vi "Server Panel.vi"(8 "error in":errorcluster, 11 "server session ref":variant) -> (0 "error out":errorcluster, 3 "server session ref out":variant)   [LabVIEW 2020]
doc: "This is panel of TWM server. When the server is running, a client can connect to the created named pipe and control some of the TWM function via the pipe. This panel must be opened to keep the server alive!"
uses:
  Server Session Reference.ctl
  Server Session.ctl
  varilib/SGUI Assign References Mode.ctl
  Server Event.ctl
  Server Client Request.ctl
  Server Event Command.ctl
  varilib/SGUI Assign Multiple Strings With Tags By Label.vi
  varilib/varilib.lvlib
panel:
  out "log panel ref":refnum<vi>
  out "log ref":refnum<vi>
  in  "btn view log":bool
  in  "Log traffic":bool
  out "srv session":T1
  out "server":i32
  in  "btn srv exit":bool
  out "str last cmd":string caption="Last command header"
  out "led run":bool caption="Running"
  in  "btn srv stop":bool
  in  "btn srv start":bool
  in  "pipe name":string="\\\\.\\pipe\\TWM:server" caption="Named Pipe Identifier"
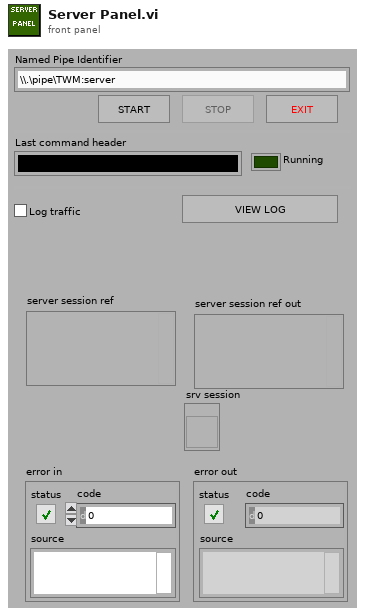
[diagram p1: front panel]
types:
  T1 = typedef "Server Session Reference.ctl" = refnum<vi>
  T2 = typedef "varilib.lvlib/SGUI Assign References Mode.ctl" = enum16{"Add to stack", "Overwrite", "Release last", "Release ID"}
  T3 = typedef "Server Session.ctl" = cluster{"cmd event":variant, "answer event":variant}
  T4 = typedef "Server Event.ctl" = cluster{"client request":T5, "command":T6}
  T5 = typedef "Server Client Request.ctl" = cluster{"info data":string, "answer handle":i32}
  T6 = typedef "Server Event Command.ctl" = enum16{"None", "Restart", "Identify", "Set measurement", "Start", "Get status", "Get result", "Stop", "Set corrections", "Get algorithm info"}
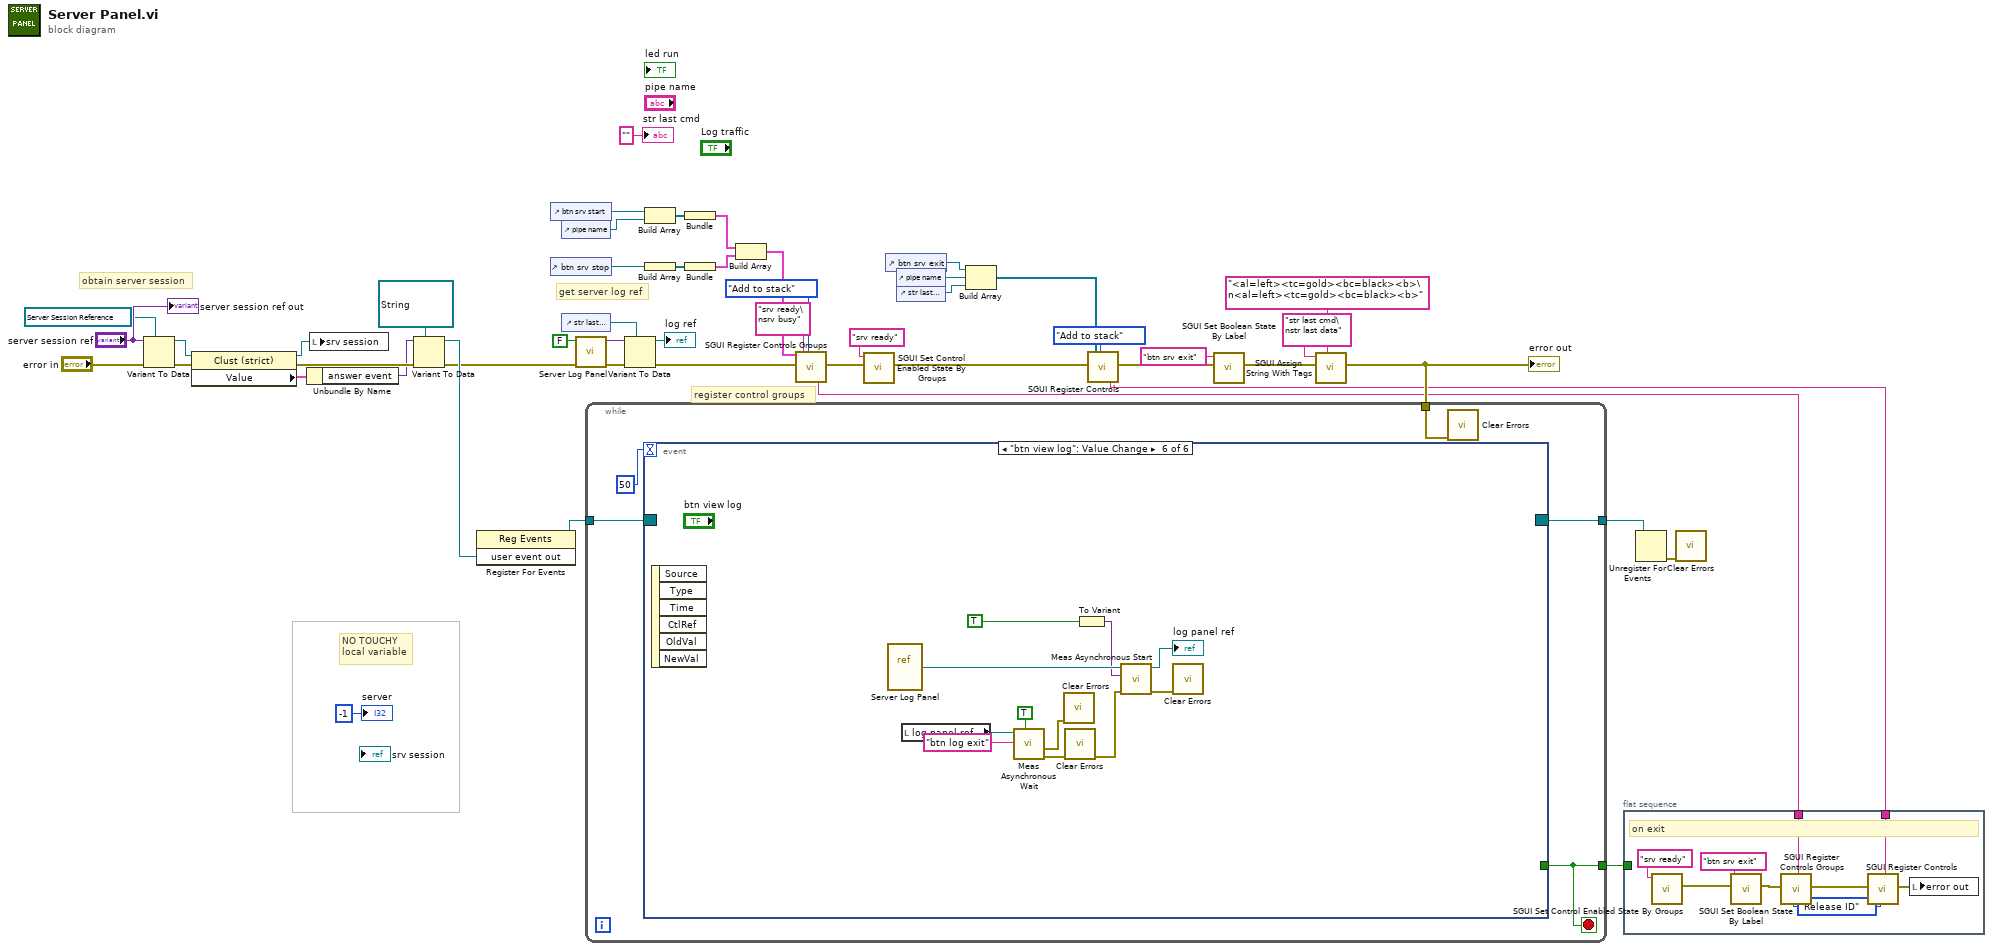
[diagram p0: block diagram]
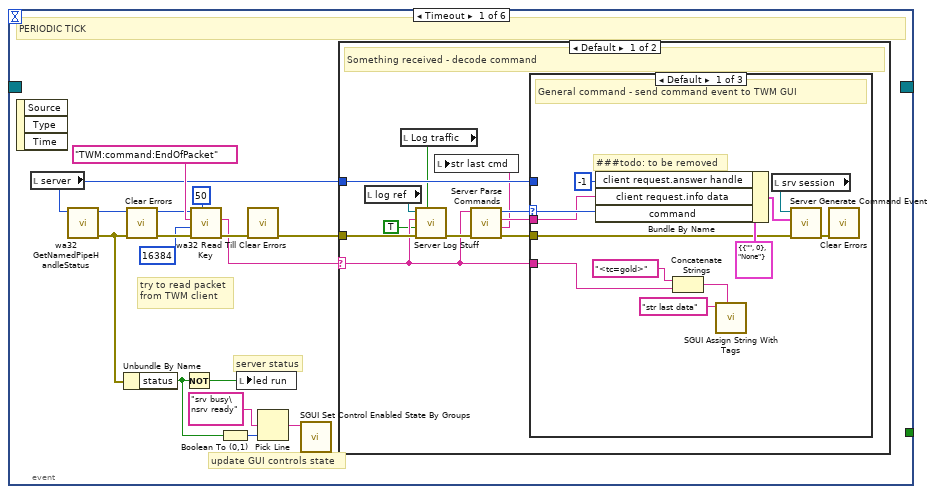
[diagram p2: hidden frame]
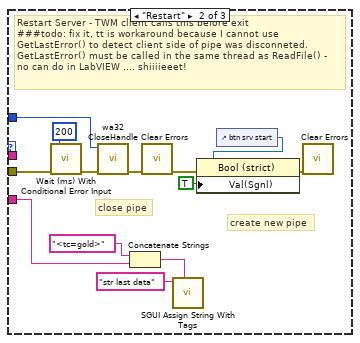
[diagram p3: hidden frame]
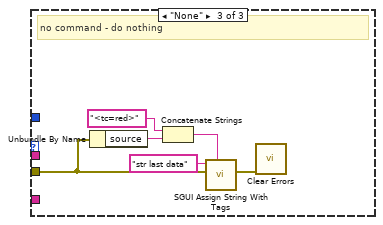
[diagram p4: hidden frame]
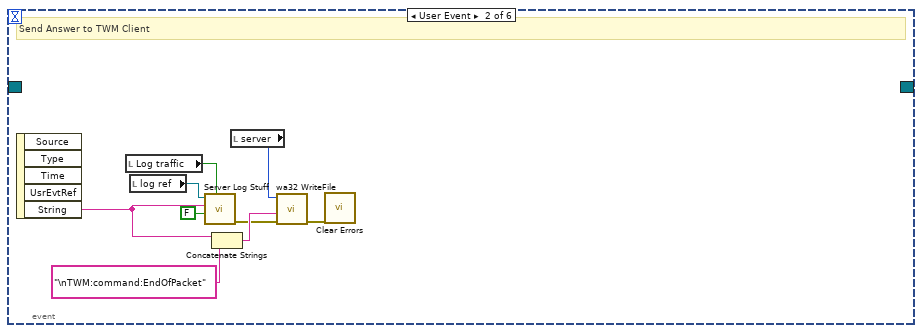
[diagram p6: hidden frame]
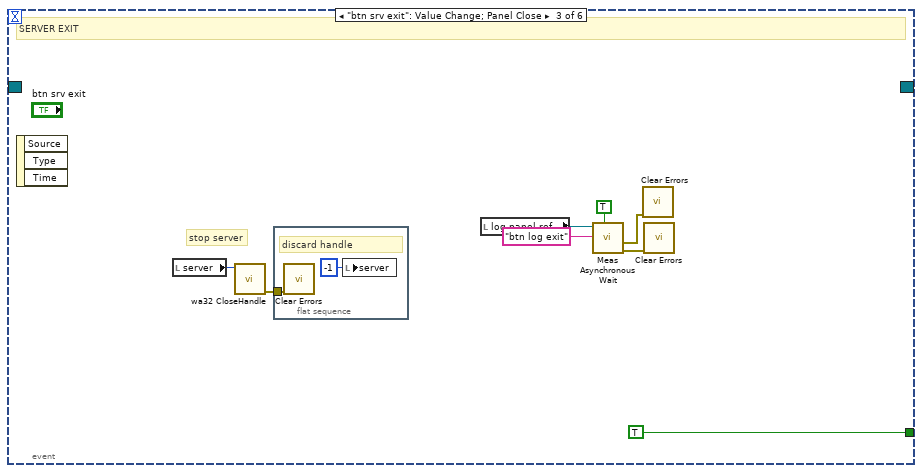
[diagram p7: hidden frame]
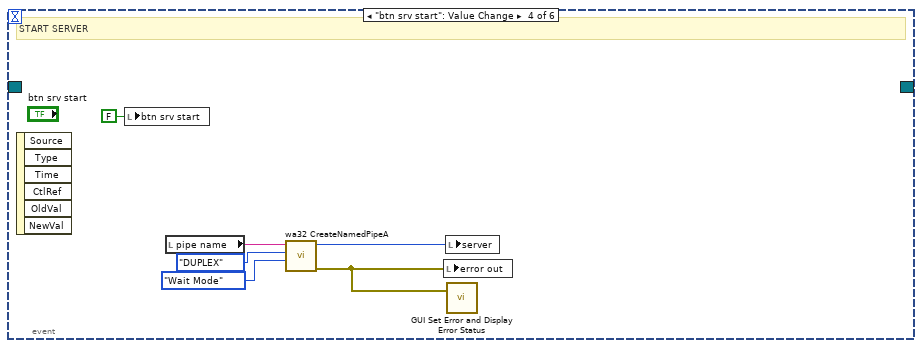
[diagram p8: hidden frame]
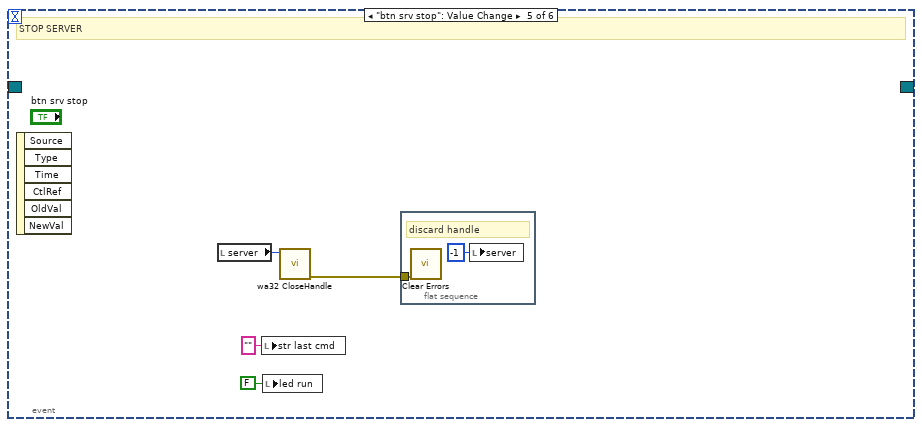
[diagram p9: hidden frame]
diagram:
  # "get server log ref"
  # "obtain server session"
  # "NO TOUCHY\nlocal variable"
  # "register control groups"
  n1 = Variant To Data(error in="error in", type=T1 refnum ("server ref"), Variant="server session ref") -> (data=w20:T1, error out=w21:errorcluster)
  n2 = property class="Clust (strict)"(reference=w20, error in=w21) -> (reference out=w19:T1, error out=w17:errorcluster, "Value"=w18:T3)
  n3 = Unbundle By Name(w18) -> ("answer event"=w16:variant)
  n4 = local write "srv session"(w19) -> ()
  n5 = Variant To Data(error in=w17, type=refnum<user-event> refnum ("user event out"), Variant=w16) -> (data=w14:refnum<user-event>, error out=w7:errorcluster)
  n6 = register-events(w14) -> (reference out=w22:refnum<event-registration>)  [unwired: 2 in, 1 out]
  n7 = control-ref of="btn srv start"() -> (w45:refnum<vi>)
  n8 = control-ref of="btn srv stop"() -> (w46:refnum<vi>)
  n9 = control-ref of="pipe name"() -> (w44:refnum<vi>)
  n10 = control-ref of="str last cmd"() -> (w2:refnum<vi>)
  n11 = call "Server Log Panel.vi"("error in"=w7, "open window (false)"=FALSE) -> ("error out"=w5:errorcluster, "text ref"=w3:variant)  [unwired: 8 in]
  n12 = Variant To Data(error in=w5, type=w2, Variant=w3) -> (data=→"log ref":refnum<vi>, error out=w4:errorcluster)
  n13 = Build Array(w45, w44) -> (w49:refnum<vi>[])
  n14 = Build Array(w46) -> (w47:refnum<vi>[])
  n15 = Bundle(w49) -> (w50:cluster{refnum<vi>[]})  [unwired: 1 in]
  n16 = Bundle(w47) -> (w48:cluster{refnum<vi>[]})  [unwired: 1 in]
  n17 = Build Array(w50, w48) -> (w43:cluster{refnum<vi>[]}[])
  n18 = call "SGUI Register Controls Groups.vi"("control groups"=w43, "error in"=w4, "groups names"="srv ready\nsrv busy", "register mode (overwrite)"=SGUI_Assign_References_Mode."Add to stack") -> ("assigned ID"=w25:string, "error out"=w40:errorcluster)  [unwired: 14 in]
  n19 = call "SGUI Set Control Enabled State By Groups.vi"("error in"=w40, "group name to enable (none)"="srv ready") -> ("error out"=w37:errorcluster)  [unwired: 8 in, 1 out]
  n20 = control-ref of="btn srv exit"() -> (w8:refnum<vi>)
  n21 = control-ref of="pipe name"() -> (w36:refnum<vi>)
  n22 = control-ref of="str last cmd"() -> (w35:refnum<vi>)
  n23 = Build Array(w8, w36, w35) -> (w34:refnum<vi>[])
  n24 = call "SGUI Register Controls.vi"("error in"=w37, "control references (empty)"=w34, "register mode (overwrite)"=SGUI_Assign_References_Mode."Add to stack") -> ("assigned ID"=w24:string, "error out"=w11:errorcluster)  [unwired: 14 in, 1 out]
  n25 = call "SGUI Set Boolean State By Label.vi"("error in"=w11, "control label(s) ('btn stop')"="btn srv exit" ("labels (empty)")) -> ("error out"=w10:errorcluster)  [unwired: 8 in, 1 out]
  n26 = call-poly "SGUI Assign String With Tags.vi"("error in"=w10, "label(s) (empty)"="str last cmd\nstr last data", "string (empty)"="<al=left><tc=gold><bc=black><b>\n<al=left><tc=gold><bc=black><b>") -> ("error out"=w30:errorcluster)  [unwired: 7 in, 1 out]
  "error out" <- w30
  n27 = while {
    tunnel: w30 -> [w54]
    tunnel: [w53] -> w38
    tunnel: w22 -> [w52]
    tunnel: [w51] -> w13
    stop <- w53 stop-if-true
    n28 = event shown="[5] \"btn view log\": Value Change" {
      selector: w52 -> [_ _ _ _ _ _]
      dyn-events: [_ _ _ _ _ _] -> w51
      timeout: 50 -> [_ _ _ _ _ _]
      tunnel: [_ _ TRUE _ _ _] -> w53
      event Timeout {
        # "try to read packet\nfrom TWM client"
        # "server status"
        # "update GUI controls state"
        # "PERIODIC TICK"
        n29 = event-data() -> ()  [unwired: 1 in, 3 out]
        n30 = local read "server"() -> (w57:i32)
        n31 = call "wa32 GetNamedPipeHandleStatus.vi"("handle"=w57) -> ("error out"=w62:errorcluster, "handle out"=w58:i32)  [unwired: 7 in, 2 out]
        n32 = Unbundle By Name(w62) -> ("status"=w64:bool)
        n33 = call <vilib>:"Clear Errors.vi"("error in (no error)"=w62) -> ("error out"=w59:errorcluster)  [unwired: 5 in, 1 out]
        n34 = Not(x=w64) -> (.not. x?=w68:bool)
        n35 = call "wa32 Read Till Key.vi"("timeout [ms] (1000)"=50, "error in"=w59, "max message length (1024)"=16384, "key string"="TWM:command:EndOfPacket", "handle"=w58) -> ("error out"=w69:errorcluster, "read message"=w61:string)  [unwired: 4 in, 1 out]
        n36 = Boolean To (0,1)(Boolean=w64) -> (0, 1=w67:i16)
        n37 = local write "led run"(w68) -> ()
        n38 = call <vilib>:"Clear Errors.vi"("error in (no error)"=w69) -> ("error out"=w60:errorcluster)  [unwired: 5 in, 1 out]
        n39 = Pick Line(multi-line string="srv busy\nsrv ready", line index=w67) -> (output string=w65:string)  [unwired: 1 in]
        n40 = call "SGUI Set Control Enabled State By Groups.vi"("group name to enable (none)"=w65) -> ()  [unwired: 9 in, 2 out]
        n41 = case shown="Default" w61 {
          selector: w61 -> [w73 _]
          tunnel: w60 -> [w76 _]
          tunnel: w57 -> [w79 _]
          frame Default {
            # "Something received - decode command"
            n42 = local read "log ref"() -> (w72:refnum<vi>)
            n43 = local read "Log traffic"() -> (w74:bool)
            n44 = call "Server Log Stuff.vi"("log (true)"=w74, "error in"=w76, "write/read (false:write)"=TRUE, "String"=w73, "log ref"=w72) -> ("error out"=w75:errorcluster)  [unwired: 6 in]
            n45 = call "Server Parse Commands.vi"("error in"=w75, "string"=w73) -> ("error out"=w80:errorcluster, "command string"=w77:string, "command data"=w78:string, "command"=w81:T6)  [unwired: 6 in]
            n46 = local write "str last cmd"(w77) -> ()
            n47 = case shown="Default" w81 {
              selector: w81 -> [w88 _ _]
              tunnel: w80 -> [w89 w101 w110]
              tunnel: w79 -> [_ w106 _]
              tunnel: w78 -> [w82 _ _]
              tunnel: w73 -> [w83 w94 _]
              frame Default {
                # "###todo: to be removed"
                # "General command - send command event to TWM GUI"
                n48 = Bundle By Name(cluster=T4 {"client request"={"info data"="", "answer handle"=0}, "command"=enum."None"} ("event data"), "client request.answer handle"=-1, "client request.info data"=w82, "command"=w88) -> (w90:T4)
                n49 = Concatenate Strings("<tc=gold>" ("string"), w83) -> (w85:string)
                n50 = call-poly "SGUI Assign String With Tags.vi"("label(s) (empty)"="str last data", "string (empty)"=w85) -> ()  [unwired: 8 in, 2 out]
                n51 = local read "srv session"() -> (w92:T1)
                n52 = call "Server Generate Command Event.vi"("error in"=w89, "event data"=w90, "server event ref"=w92) -> ("error out"=w93:errorcluster)  [unwired: 8 in]
                n53 = call <vilib>:"Clear Errors.vi"("error in (no error)"=w93) -> ()  [unwired: 5 in, 2 out]
              }
              frame "Restart" {
                # "create new pipe"
                # "close pipe"
                # "Restart Server - TWM client calls this before exit\n###todo: fix it, tt is workaround because I cannot use\nGetLastError() to detect client side of pipe was disconneted.\nGetLastError() must be called in the same thread as ReadFile() - \nno can do in LabVIEW .... shiiiieeet!"
                n54 = call "Wait (ms) With Conditional Error Input.vi"("error in (no error)"=w101, "milliseconds to wait"=u32 200) -> ("error out"=w100:errorcluster)  [unwired: 8 in, 1 out]
                n55 = call "wa32 CloseHandle.vi"("error in"=w100, "handle"=w106) -> ("error out"=w105:errorcluster)  [unwired: 9 in]
                n56 = Concatenate Strings("<tc=gold>" ("string"), w94) -> (w96:string)
                n57 = call <vilib>:"Clear Errors.vi"("error in (no error)"=w105) -> ("error out"=w98:errorcluster)  [unwired: 5 in, 1 out]
                n58 = call-poly "SGUI Assign String With Tags.vi"("label(s) (empty)"="str last data", "string (empty)"=w96) -> ()  [unwired: 8 in, 2 out]
                n59 = control-ref of="btn srv start"() -> (w104:refnum<vi>)
                n60 = property class="Bool (strict)"(reference=w104, error in=w98, "Val(Sgnl)"=TRUE) -> (error out=w102:errorcluster)  [unwired: 1 out]
                n61 = call <vilib>:"Clear Errors.vi"("error in (no error)"=w102) -> ()  [unwired: 5 in, 2 out]
              }
              frame "None" {
                # "no command - do nothing"
                n62 = Unbundle By Name(w110) -> ("source"=w109:string)
                n63 = Concatenate Strings("<tc=red>" ("string"), w109) -> (w108:string)
                n64 = call-poly "SGUI Assign String With Tags.vi"("error in"=w110, "label(s) (empty)"="str last data", "string (empty)"=w108) -> ("error out"=w112:errorcluster)  [unwired: 7 in, 1 out]
                n65 = call <vilib>:"Clear Errors.vi"("error in (no error)"=w112) -> ()  [unwired: 5 in, 2 out]
              }
            }
          }
          frame "" {
          }
        }
      }
      event User Event {
        # "Send Answer to TWM Client"
        n66 = event-data() -> ("String"=w116:string)  [unwired: 1 in, 4 out]
        n67 = local read "Log traffic"() -> (w115:bool)
        n68 = local read "log ref"() -> (w114:refnum<vi>)
        n69 = call "Server Log Stuff.vi"("log (true)"=w115, "write/read (false:write)"=FALSE, "String"=w116, "log ref"=w114) -> ("error out"=w117:errorcluster)  [unwired: 7 in]
        n70 = Concatenate Strings(w116, "\nTWM:command:EndOfPacket" ("key string")) -> (w119:string)
        n71 = local read "server"() -> (w121:i32)
        n72 = call "wa32 WriteFile.vi"("error in"=w117, "string data (empty)"=w119, "handle"=w121) -> ("error out"=w118:errorcluster)  [unwired: 6 in, 2 out]
        n73 = call <vilib>:"Clear Errors.vi"("error in (no error)"=w118) -> ()  [unwired: 5 in, 2 out]
      }
      event "btn srv exit": Value Change; Panel Close {
        # "stop server"
        # "SERVER EXIT"
        n74 = event-data() -> ()  [unwired: 1 in, 3 out]
        n75 = local read "server"() -> (w128:i32)
        n76 = call "wa32 CloseHandle.vi"("handle"=w128) -> ("error out"=w127:errorcluster)  [unwired: 10 in]
        n77 = flat-sequence {
          tunnel: w127 -> [w131]
          frame #0 {
            # "discard handle"
            n78 = call <vilib>:"Clear Errors.vi"("error in (no error)"=w131) -> ()  [unwired: 5 in, 2 out]
            n79 = local write "server"(-1 ("server")) -> ()
          }
        }
        n80 = local read "log panel ref"() -> (w126:refnum<vi>)
        n81 = call "Meas Asynchronous Wait.vi"("Wait for exit? (False)"=TRUE, "stop button name ('btn stop')"="btn log exit", "VI reference (empty)"=w126) -> ("error out"=w123:errorcluster, "VI's error out"=w122:errorcluster)  [unwired: 4 in, 3 out]
        n82 = call <vilib>:"Clear Errors.vi"("error in (no error)"=w122) -> ()  [unwired: 5 in, 2 out]
        n83 = call <vilib>:"Clear Errors.vi"("error in (no error)"=w123) -> ()  [unwired: 5 in, 2 out]
      }
      event "btn srv start": Value Change {
        # "START SERVER"
        n84 = event-data() -> ()  [unwired: 1 in, 6 out]
        n85 = local write "btn srv start"(FALSE ("btn srv start")) -> ()
        n86 = local read "pipe name"() -> (w137:string)
        n87 = call "wa32 CreateNamedPipeA.vi"("pipe mode"=enum16{"Wait Mode", "No Wait Mode"}."Wait Mode", "open mode"=enum16{"INBOUND", "OUTBOUND", "DUPLEX"}."DUPLEX", "file path"=w137) -> ("error out"=w133:errorcluster, "handle"=w134:i32)  [unwired: 7 in]
        n88 = local write "error out"(w133) -> ()
        n89 = local write "server"(w134) -> ()
        n90 = call "GUI Set Error and Display Error Status.vi"("error in"=w133) -> ()  [unwired: 4 in]
      }
      event "btn srv stop": Value Change {
        # "STOP SERVER"
        n91 = event-data() -> ()  [unwired: 1 in, 6 out]
        n92 = local read "server"() -> (w141:i32)
        n93 = local write "str last cmd"("" ("str last cmd")) -> ()
        n94 = local write "led run"(FALSE ("led run")) -> ()
        n95 = call "wa32 CloseHandle.vi"("handle"=w141) -> ("error out"=w140:errorcluster)  [unwired: 10 in]
        n96 = flat-sequence {
          tunnel: w140 -> [w143]
          frame #0 {
            # "discard handle"
            n97 = call <vilib>:"Clear Errors.vi"("error in (no error)"=w143) -> ()  [unwired: 5 in, 2 out]
            n98 = local write "server"(-1 ("server")) -> ()
          }
        }
      }
      event "btn view log": Value Change {
        n99 = event-data() -> ()  [unwired: 1 in, 6 out]
        n100 = vi-ref "Server Log Panel.vi"() -> (w153:refnum<vi>)
        n101 = local read "log panel ref"() -> (w149:refnum<vi>)
        n102 = call "Meas Asynchronous Wait.vi"("Wait for exit? (False)"=TRUE, "stop button name ('btn stop')"="btn log exit", "VI reference (empty)"=w149) -> ("error out"=w146:errorcluster, "VI's error out"=w145:errorcluster)  [unwired: 4 in, 3 out]
        n103 = call <vilib>:"Clear Errors.vi"("error in (no error)"=w145) -> ()  [unwired: 5 in, 2 out]
        n104 = call <vilib>:"Clear Errors.vi"("error in (no error)"=w146) -> ("error out"=w144:errorcluster)  [unwired: 5 in, 1 out]
        n105 = To Variant(anything=TRUE) -> (Variant=w151:variant)
        n106 = call "Meas Asynchronous Start.vi"("error in"=w144, "parameter in"=w151, "Static VI reference in (empty)"=w153) -> ("error out"=w154:errorcluster, "async VI reference out"=→"log panel ref":refnum<vi>)  [unwired: 7 in]
        n107 = call <vilib>:"Clear Errors.vi"("error in (no error)"=w154) -> ()  [unwired: 5 in, 2 out]
      }
    }
    n108 = call <vilib>:"Clear Errors.vi"("error in (no error)"=w54) -> ()  [unwired: 5 in, 2 out]
  }
  n109 = flat-sequence {
    tunnel: w38 -> [_]
    tunnel: w25 -> [w159]
    tunnel: w24 -> [w158]
    frame #0 {
      w160 = SGUI_Assign_References_Mode."Release ID" ("register mode (overwrite)")
      # "on exit"
      n110 = call "SGUI Set Control Enabled State By Groups.vi"("group name to enable (none)"="srv ready") -> ("error out"=w156:errorcluster)  [unwired: 9 in, 1 out]
      n111 = call "SGUI Set Boolean State By Label.vi"("error in"=w156, "control label(s) ('btn stop')"="btn srv exit" ("labels (empty)")) -> ("error out"=w155:errorcluster)  [unwired: 8 in, 1 out]
      n112 = call "SGUI Register Controls Groups.vi"("error in"=w155, "register mode (overwrite)"=w160, "controls ID (empty)"=w159) -> ("error out"=w162:errorcluster)  [unwired: 15 in, 1 out]
      n113 = call "SGUI Register Controls.vi"("error in"=w162, "register mode (overwrite)"=w160, "controls ID (empty)"=w158) -> ("error out"=w161:errorcluster)  [unwired: 14 in, 2 out]
      n114 = local write "error out"(w161) -> ()
    }
  }
  n115 = Unregister For Events(event registration refnum=w13) -> (error out=w12:errorcluster)  [unwired: 1 in]
  n116 = call <vilib>:"Clear Errors.vi"("error in (no error)"=w12) -> ()  [unwired: 5 in, 2 out]
  "str last cmd" <- "" ("str last cmd")
  "server" <- -1 ("server")
  "server session ref out" <- "server session ref"
